vi "multiply.vi"(8 "error in (no error)":errorcluster, 9 "factor image":refnum<class "Image.lvclass">, 10 "factor":dbl=1.0, 11 "Image in":refnum<class "Image.lvclass">) -> (0 "error out":errorcluster, 3 "Image out":refnum<class "Image.lvclass">)   [LabVIEW 2010, in "Image.lvclass"]
uses:
  Image.lvclass
  storage_mode.ctl
  ErrorController/ErrorController/class_data.vi
  <vilib>/vision/NI_Vision_Development_Module.lvlib
  ErrorController/ErrorController/ErrorController.lvclass
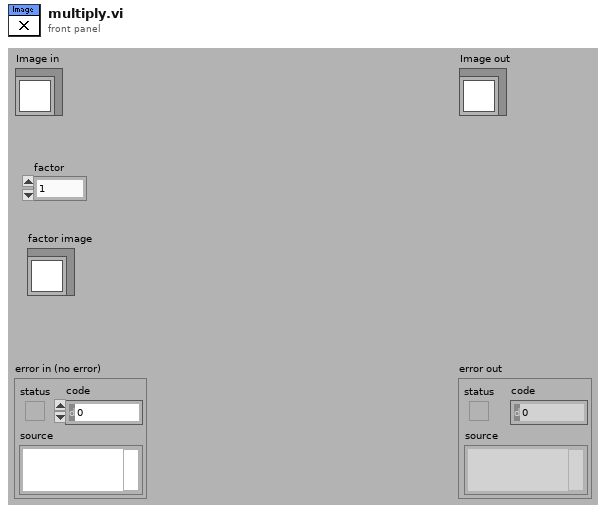
[diagram p1: front panel]
types:
  T1 = typedef "Image.lvclass/storage_mode.ctl" = enum16{"RAM", "disk"}
  T2 = typedef "IMAQ Image.ctl" = refnum<image>
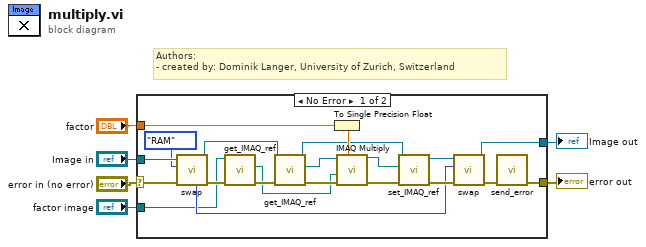
[diagram p0: block diagram]
diagram:
  # "Authors: \n- created by: Dominik Langer, University of Zurich, Switzerland"
  n1 = case shown="No Error" "error in (no error)" {
    selector: "error in (no error)" -> [w18 w29]
    tunnel: [w7 w29] -> w5
    tunnel: [w20 w28] -> w3
    tunnel: "Image in" -> [w21 w28]
    tunnel: "factor" -> [w27 _]
    tunnel: "factor image" -> [w10 _]
    frame No Error {
      n2 = call-dynamic "swap.vi"("error in (no error)"=w18, "storage type target"=storage_mode."RAM", "Image in"=w21) -> ("error out"=w13:errorcluster, "Image out"=w11:refnum<class "Image.lvclass">, "previous storage mode"=w15:T1)  [unwired: 6 out]
      n3 = call-dynamic "get_IMAQ_ref.vi"("error in (no error)"=w13, "Image.lvclass in"=w10) -> ("error out"=w12:errorcluster, "Image"=w9:T2)  [unwired: 8 out]
      n4 = call-dynamic "get_IMAQ_ref.vi"("error in (no error)"=w12, "Image.lvclass in"=w11) -> ("error out"=w17:errorcluster, "Image"=w24:T2, "Image.lvclass out"=w23:refnum<class "Image.lvclass">)  [unwired: 7 out]
      n5 = To Single Precision Float(number=w27) -> (single precision float=w26:sgl)
      n6 = call "IMAQ Multiply"("Image Src A"=w24, "Constant"=w26, "Image Src B"=w9, "error in (no error)"=w17) -> ("Image Dst Out"=w25:T2, "error out"=w16:errorcluster)  [unwired: 1 in, 2 out]
      n7 = call-dynamic "set_IMAQ_ref.vi"("error in (no error)"=w16, "Image"=w25, "Image.lvclass in"=w23) -> ("error out"=w19:errorcluster, "Image.lvclass out"=w22:refnum<class "Image.lvclass">)  [unwired: 7 out]
      n8 = call-dynamic "swap.vi"("error in (no error)"=w19, "storage type target"=w15, "Image in"=w22) -> ("error out"=w8:errorcluster, "Image out"=w20:refnum<class "Image.lvclass">)  [unwired: 7 out]
      n9 = call "send_error.vi"("error in (no error)"=w8) -> ("error out"=w7:errorcluster)  [unwired: 10 in]
    }
    frame Error {
    }
  }
  "error out" <- w5
  "Image out" <- w3
